vi "Main.vi"() -> ()   [LabVIEW 2014]
uses:
  TypeDefs/Errors.ctl
  <vilib>/Utility/file.llb/Read From Spreadsheet File (string).vi
  <vilib>/Waveform/DWDTOps.llb/DWDT Analog to Digital.vi
panel:
  out "Array":dbl[](array[numeric])
  out "Array 3":dbl[](array[numeric])
  out "Digital signals":cluster{dbl[], dbl[]}[](graph)
  out "digitsl signals":cluster{dbl[], dbl[]}(graph)
  in  "# of Files":i32=10
  out "# of rows":i32
  in  "File Locations":T1={"01 File Path"=path "C:/Users/502424328/Desktop/Ex Dish Inverter Board Data.csv", "02 File Path"=path "C:/Users/502424328/Desktop/Ex Dish Inverter Board Data.csv", "03 File Path"=path "C:/Users/502424328/Desktop/Ex Dish Inverter Board Data.csv", "04 File Path"=path "C:/Users/502424328/Desktop/Ex Dish Inverter Board Data.csv", "05 File Path"=path "C:/Users/502424328/Desktop/Ex Dish Inverter Board Data.csv", "06 File Path"=path "C:/Users/502424328/Desktop/Ex Dish Inverter Board Data.csv", "07 File Path"=path "C:/Users/502424328/Desktop/Ex Dish Inverter Board Data.csv", "08 File Path"=path "C:/Users/502424328/Desktop/Ex Dish Inverter Board Data.csv", "09 File Path"=path "C:/Users/502424328/Desktop/Ex Dish Inverter Board Data.csv", "10 File Path"=path "C:/Users/502424328/Desktop/Ex Dish Inverter Board Data.csv"}
  in  "Tab Control":T2(tab)
  out "Current (mA)":cluster{dbl[], dbl[]}(graph)
  out "Motor Type\n0 = MAIN\n1 = DRAIN":digitalwaveform(graph)
  out "XY Graph 10":cluster{dbl[], dbl[]}[](graph)
  out "Errors 1":T3
  out "XY Graph 9":cluster{dbl[], dbl[]}[](graph)
  out "Motor Type 2\n0 = MAIN\n1 = DRAIN 2":digitalwaveform(graph)
  out "Errors 2":T3
  out "Current 2 (mA)":cluster{dbl[], dbl[]}(graph)
  out "XY Graph 8":cluster{dbl[], dbl[]}[](graph)
  out "Motor Type 3\n0 = MAIN\n1 = DRAIN":digitalwaveform(graph)
  out "Errors 3":T3
  out "Current 3 (mA)":cluster{dbl[], dbl[]}(graph)
  out "XY Graph 7":cluster{dbl[], dbl[]}[](graph)
  out "Motor Type 4\n0 = MAIN\n1 = DRAIN":digitalwaveform(graph)
  out "Errors 4":T3
  out "Current 4 (mA)":cluster{dbl[], dbl[]}(graph)
  out "XY Graph 6":cluster{dbl[], dbl[]}[](graph)
  out "Motor Type 5\n0 = MAIN\n1 = DRAIN":digitalwaveform(graph)
  out "Errors 5":T3
  out "Current 5 (mA)":cluster{dbl[], dbl[]}(graph)
  out "Motor Type 6\n0 = MAIN\n1 = DRAIN":digitalwaveform(graph)
  out "Errors 6":T3
  out "Current 6 (mA)":cluster{dbl[], dbl[]}(graph)
  out "XY Graph 5":cluster{dbl[], dbl[]}[](graph)
  out "XY Graph 4":cluster{dbl[], dbl[]}[](graph)
  out "Motor Type 7\n0 = MAIN\n1 = DRAIN":digitalwaveform(graph)
  out "Errors 7":T3
  out "Current 7 (mA)":cluster{dbl[], dbl[]}(graph)
  out "XY Graph 3":cluster{dbl[], dbl[]}[](graph)
  out "Motor Type 8\n0 = MAIN\n1 = DRAIN":digitalwaveform(graph)
  out "Errors 8":T3
  out "Current 8 (mA)":cluster{dbl[], dbl[]}(graph)
  out "XY Graph 2":cluster{dbl[], dbl[]}[](graph)
  out "Motor Type 9\n0 = MAIN\n1 = DRAIN":digitalwaveform(graph)
  out "Errors 9":T3
  out "Current 9 (mA)":cluster{dbl[], dbl[]}(graph)
  out "XY Graph":cluster{dbl[], dbl[]}[](graph)
  out "Motor Type 10\n0 = MAIN\n1 = DRAIN":digitalwaveform(graph)
  out "Errors 10":T3
  out "Current 10 (mA)":cluster{dbl[], dbl[]}(graph)
  out "subarray":string[][](array[string])
  out "subarray 3":string[](array[string])
  in  "stop":bool
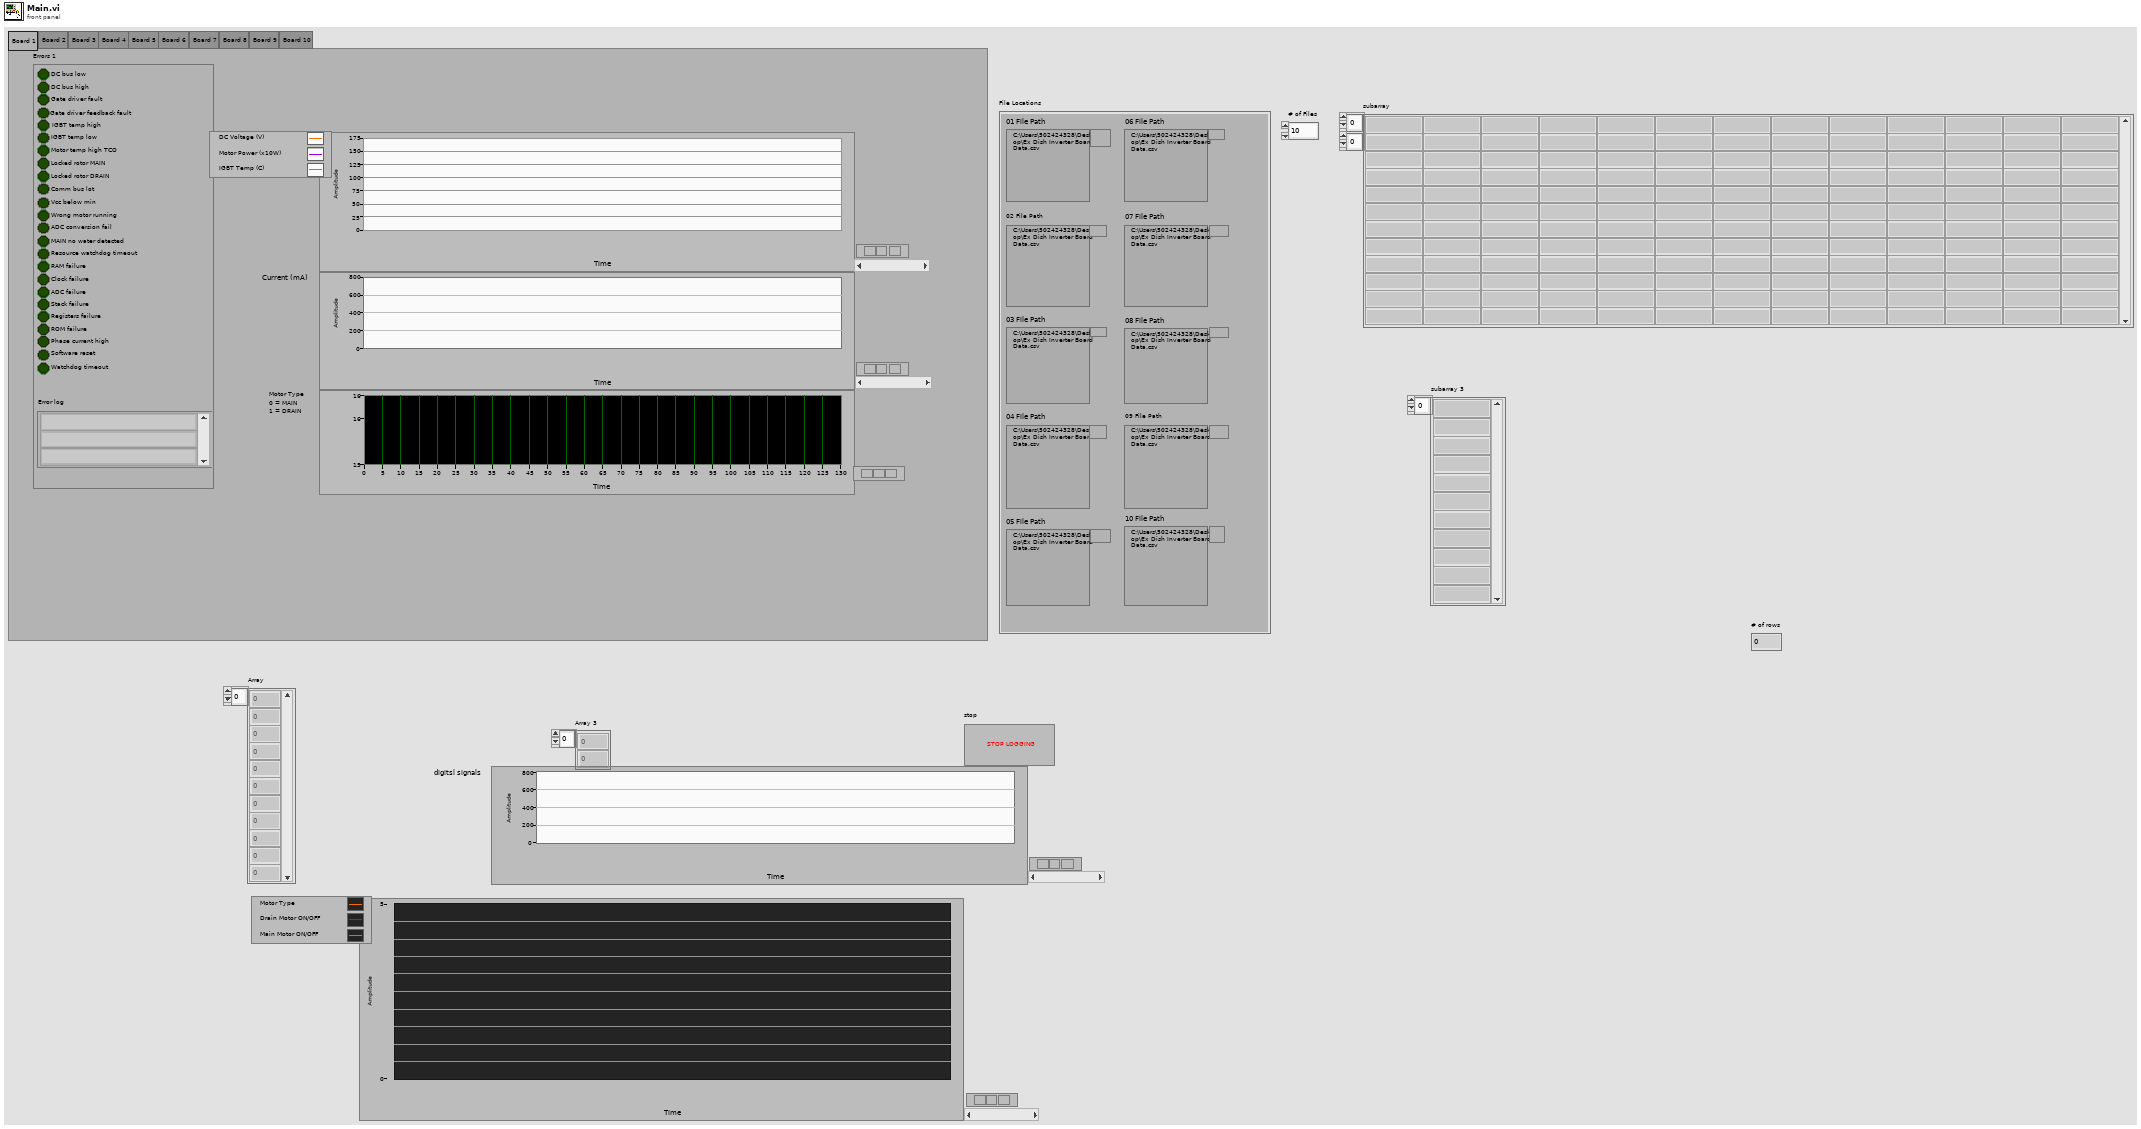
[diagram p1: front panel]
types:
  T1 = cluster{"01 File Path":path, "02 File Path":path, "03 File Path":path, "04 File Path":path, "05 File Path":path, "06 File Path":path, "07 File Path":path, "08 File Path":path, "09 File Path":path, "10 File Path":path}
  T2 = enum32{"Board 1", "Board 2", "Board 3", "Board 4", "Board 5", "Board 6", "Board 7", "Board 8", "Board 9", "Board 10"}
  T3 = typedef "Errors.ctl" = cluster{"DC bus low":bool, "DC bus high":bool, "Gate driver fault":bool, "Gate driver feedback fault":bool, "IGBT temp high":bool, "IGBT temp low":bool, "Motor temp high TCO":bool, "Locked rotor MAIN":bool, "Locked rotor DRAIN":bool, "Comm bus lot":bool, "Vcc below min":bool, "Wrong motor running":bool, "ADC conversion fail":bool, "MAIN no water detected":bool, "Resource watchdog timeout":bool, "RAM failure":bool, "Clock failure":bool, "ADC failure":bool, "Stack failure":bool, "Registers failure":bool, "ROM failure":bool, "Phase current high":bool, "Software reset":bool, "Watchdog timeout":bool, "Error log":string[]}
  T4 = cluster{"DC Bus Voltage":dbl, "Current RMS":dbl, "Motor Power":dbl, "IGBT Temp":u16, "Motor Type":u16, "Motor Power Sign":string, "Relay Position":u16, "ADC Count":dbl, "Recirculation Motor ON/OFF":u16, "Drain Motor ON/OFF":u16}
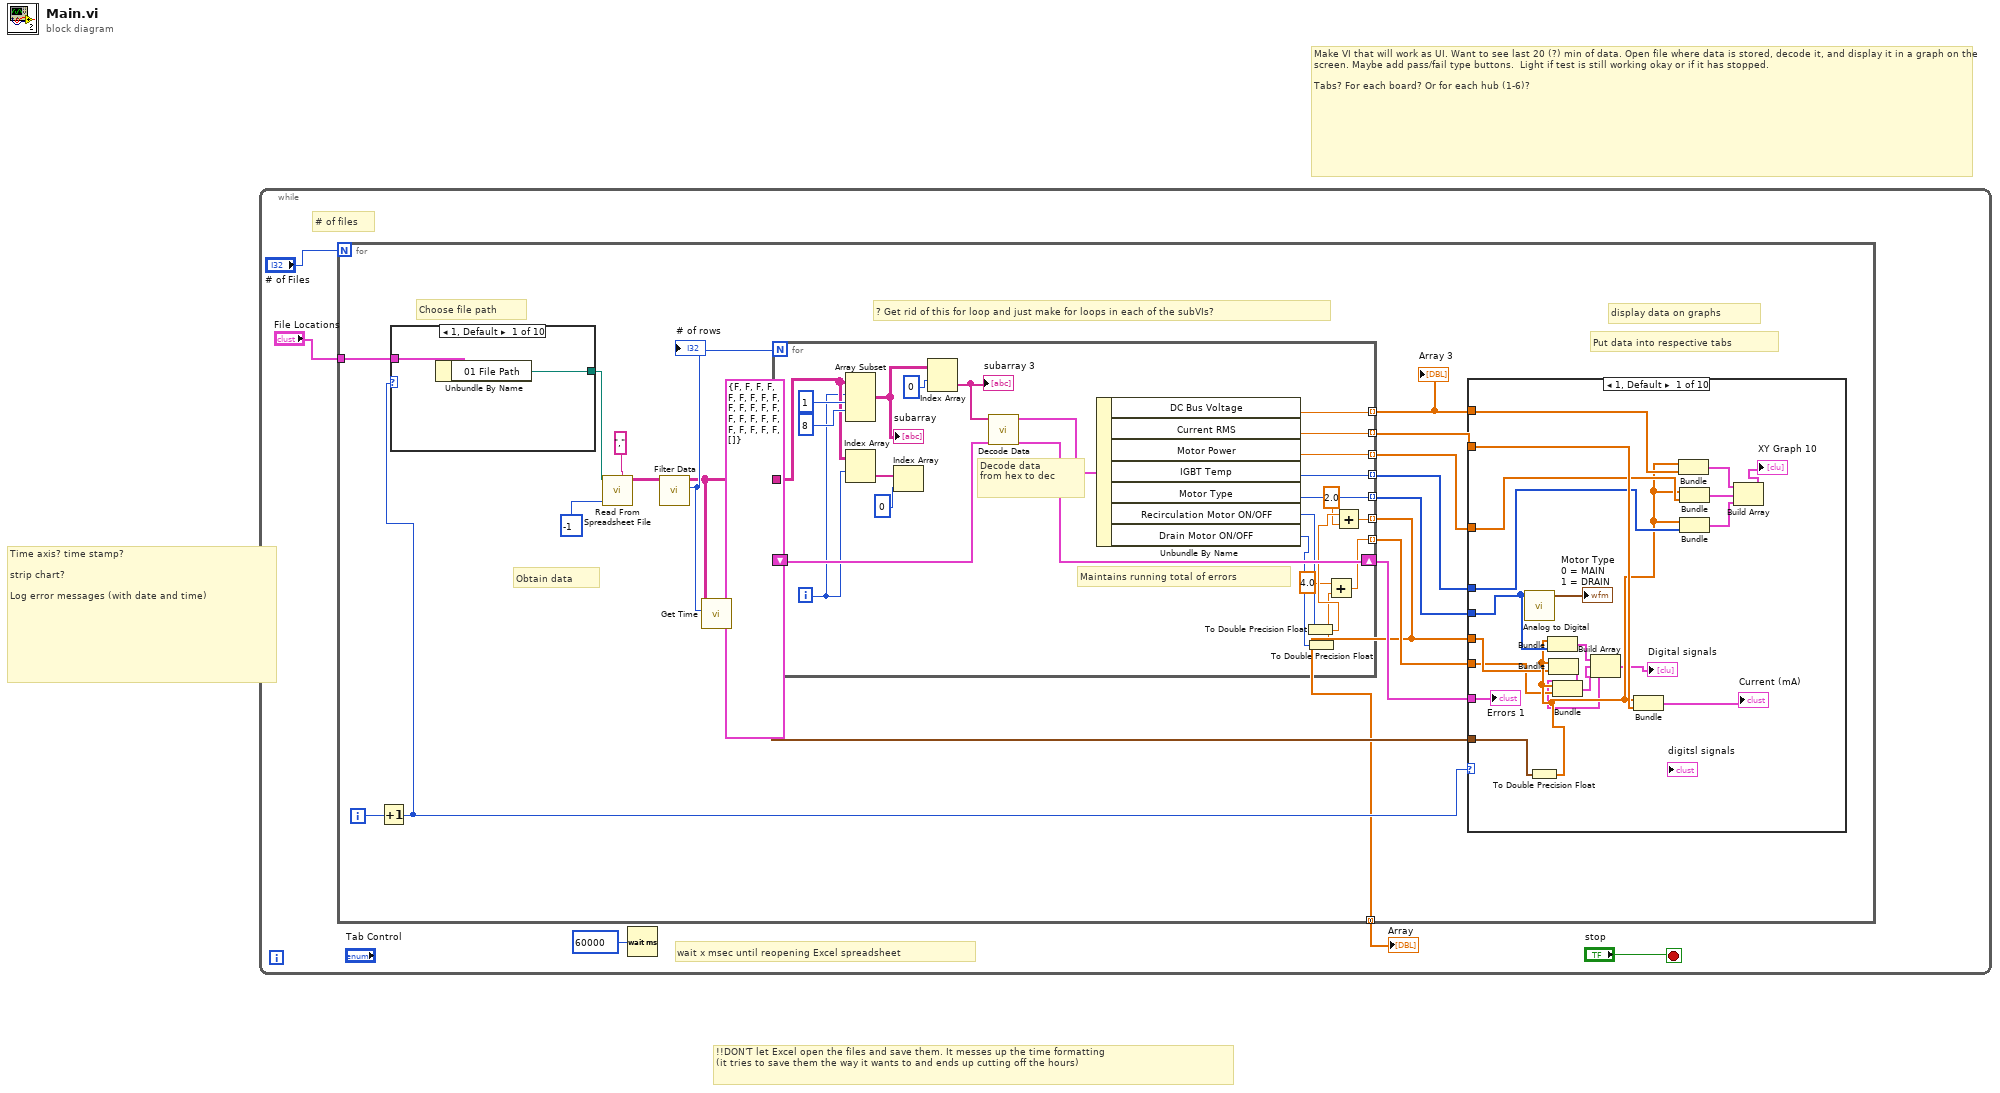
[diagram p0: block diagram]
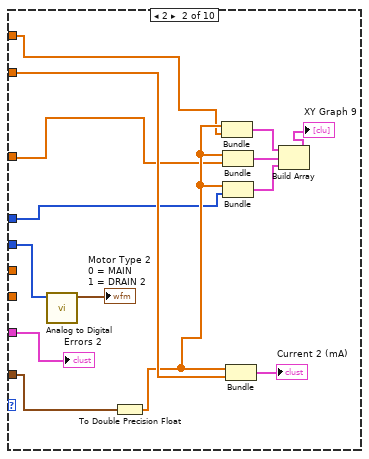
[diagram p2: hidden frame]
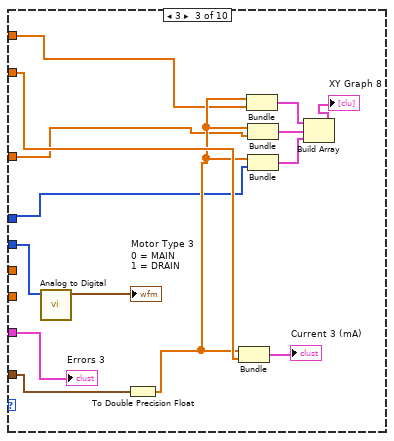
[diagram p3: hidden frame]
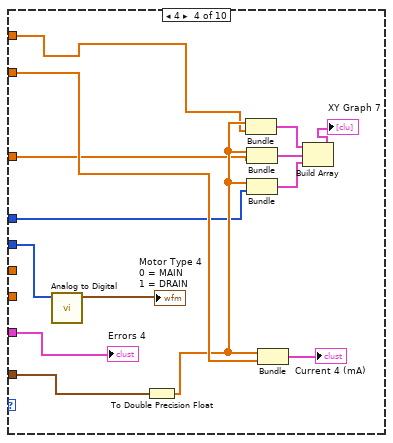
[diagram p4: hidden frame]
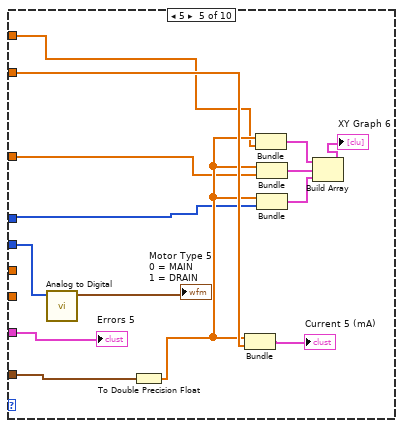
[diagram p5: hidden frame]
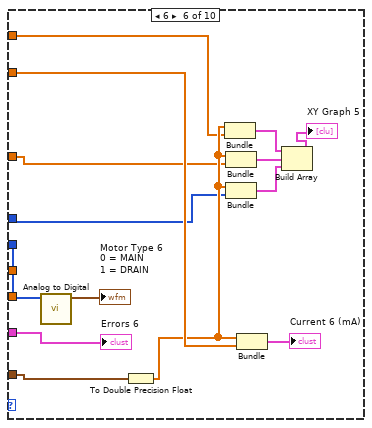
[diagram p6: hidden frame]
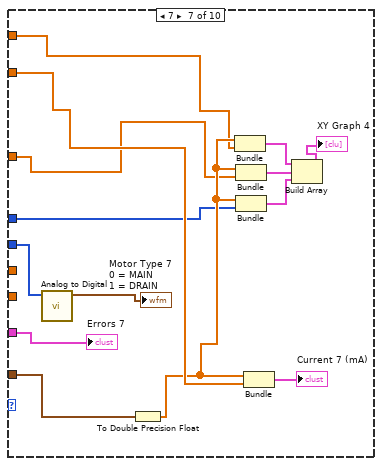
[diagram p7: hidden frame]
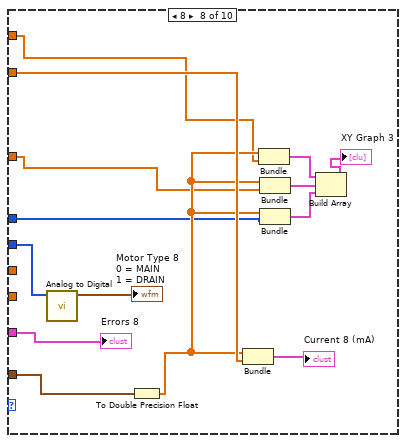
[diagram p8: hidden frame]
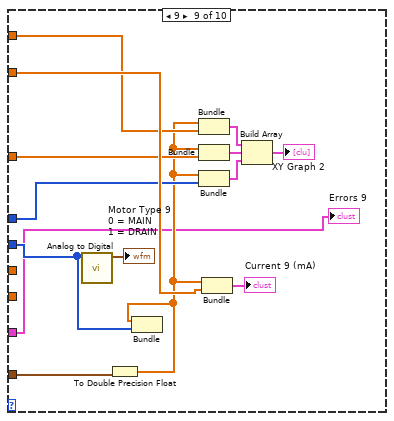
[diagram p9: hidden frame]
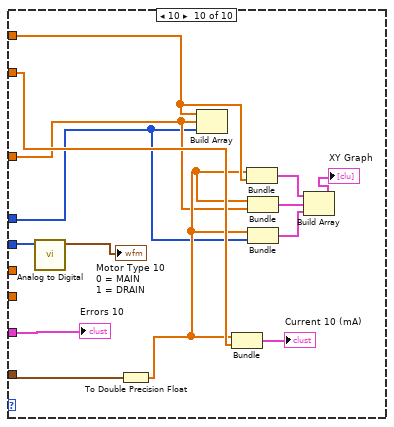
[diagram p10: hidden frame]
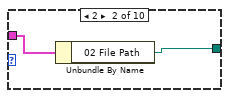
[diagram p11: hidden frame]
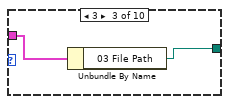
[diagram p12: hidden frame]
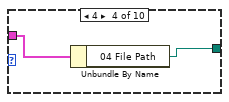
[diagram p13: hidden frame]
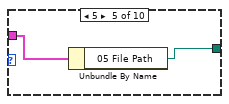
[diagram p14: hidden frame]
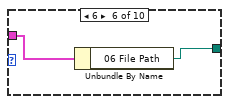
[diagram p15: hidden frame]
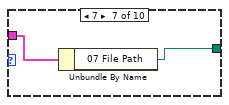
[diagram p16: hidden frame]
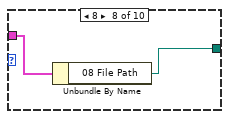
[diagram p17: hidden frame]
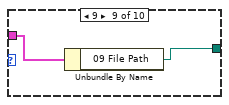
[diagram p18: hidden frame]
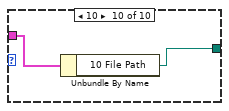
[diagram p19: hidden frame]
diagram:
  # "Time axis? time stamp?\n\nstrip chart?\n\nLog error messages (with date and time)"
  # "!!DON'T let Excel open the files and save them. It messes up the time formatting \n(it tries to save them the way it wants to and ends up cutting off the hours)"
  # "Make VI that will work as UI. Want to see last 20 (?) min of data. Open file where data is stored, decode it, and display it in a graph on the screen. Maybe add pass/fail type buttons.  Light if test is still working okay or if it has stopped. \n\nTabs? For each board? Or for each hub (1-6)?"
  n1 = while {
    stop <- "stop" stop-if-true
    # "# of files"
    # "wait x msec until reopening Excel spreadsheet"
    n2 = for {
      N: "# of Files" -> [_]
      tunnel: "File Locations" -> [w22]
      tunnel: [w6] -> w1 mode=concatenating
      i -> [w20]
      # "? Get rid of this for loop and just make for loops in each of the subVIs?"
      # "display data on graphs"
      # "Put data into respective tabs"
      # "Obtain data"
      # "Choose file path"
      n3 = Increment(x=w20) -> (x+1=w19:i32)
      n4 = case shown="1, Default" w19 {
        tunnel: w22 -> [w172 w174 w176 w178 w180 w182 w184 w186 w188 w190]
        tunnel: [w171 w173 w175 w177 w179 w181 w183 w185 w187 w189] -> w21
        frame 1, Default {
          n5 = Unbundle By Name(w172) -> ("01 File Path"=w171:path)
        }
        frame 2 {
          n6 = Unbundle By Name(w174) -> ("02 File Path"=w173:path)
        }
        frame 3 {
          n7 = Unbundle By Name(w176) -> ("03 File Path"=w175:path)
        }
        frame 4 {
          n8 = Unbundle By Name(w178) -> ("04 File Path"=w177:path)
        }
        frame 5 {
          n9 = Unbundle By Name(w180) -> ("05 File Path"=w179:path)
        }
        frame 6 {
          n10 = Unbundle By Name(w182) -> ("06 File Path"=w181:path)
        }
        frame 7 {
          n11 = Unbundle By Name(w184) -> ("07 File Path"=w183:path)
        }
        frame 8 {
          n12 = Unbundle By Name(w186) -> ("08 File Path"=w185:path)
        }
        frame 9 {
          n13 = Unbundle By Name(w188) -> ("09 File Path"=w187:path)
        }
        frame 10 {
          n14 = Unbundle By Name(w190) -> ("10 File Path"=w189:path)
        }
      }
      n15 = call-poly <vilib>:"Read From Spreadsheet File.vi"("delimiter (\\t)"="," ("delimiter (\\t)"), "number of rows (all:-1)"=-1, "file path (dialog if empty)"=w21) -> ("all rows"=w12:string[][])  [unwired: 4 in, 4 out]
      n16 = call "Filter Data.vi"("All Rows"=w12) -> ("element"=w11:i32, "new array"=w10:string[][])  [unwired: 9 in]
      "# of rows" <- w11
      n17 = call "Get Time.vi"("# of rows"=w11, "Data row"=w10) -> ("Time array"=w9:timestamp[])  [unwired: 9 in]
      n18 = for {
        N: w11 -> [_]
        tunnel: [w211] -> w16 mode=indexing
        tunnel: [w210] -> w18 mode=indexing
        tunnel: [w209] -> w17 mode=indexing
        tunnel: [w208] -> w15 mode=indexing
        tunnel: [w207] -> w14 mode=indexing
        shift-right: [w206] -> w13
        shift-left: T3 {"DC bus low"=FALSE, "DC bus high"=FALSE, "Gate driver fault"=FALSE, "Gate driver feedback fault"=FALSE, "IGBT temp high"=FALSE, "IGBT temp low"=FALSE, "Motor temp high TCO"=FALSE, "Locked rotor MAIN"=FALSE, "Locked rotor DRAIN"=FALSE, "Comm bus lot"=FALSE, "Vcc below min"=FALSE, "Wrong motor running"=FALSE, "ADC conversion fail"=FALSE, "MAIN no water detected"=FALSE, "Resource watchdog timeout"=FALSE, "RAM failure"=FALSE, "Clock failure"=FALSE, "ADC failure"=FALSE, "Stack failure"=FALSE, "Registers failure"=FALSE, "ROM failure"=FALSE, "Phase current high"=FALSE, "Software reset"=FALSE, "Watchdog timeout"=FALSE, "Error log"=[]} ("Errors Out") -> [w205]
        tunnel: w10 -> [w202]
        tunnel: [w198] -> w6 mode=indexing
        tunnel: [w197] -> w7 mode=indexing
        i -> [w199]
        # "Maintains running total of errors"
        # "Decode data\nfrom hex to dec"
        n19 = Array Subset(array=w202, index (row)=w199, length (row)=1 ("length"), index (col)=8 ("index")) -> (w213:string[][])  [unwired: 1 in]
        "subarray" <- w213
        n20 = Index Array(array=w202, index (row)=w199) -> (element=w201:string[])  [unwired: 1 in]
        n21 = Index Array(array=w201, index=0) -> ()  [unwired: 1 out]
        n22 = Index Array(array=w213, index (row)=0 ("disabled index (col)")) -> (element=w203:string[])  [unwired: 1 in]
        "subarray 3" <- w203
        n23 = call "Decode Data.vi"("Errors In"=w205, "Data Array"=w203) -> ("Errors Out"=w206:T3, "logData Out"=w204:T4)  [unwired: 8 in]
        n24 = Unbundle By Name(w204) -> ("DC Bus Voltage"=w211:dbl, "Current RMS"=w210:dbl, "Motor Power"=w209:dbl, "IGBT Temp"=w208:u16, "Motor Type"=w207:u16, "Recirculation Motor ON/OFF"=w196:u16, "Drain Motor ON/OFF"=w193:u16)
        n25 = To Double Precision Float(number=w196) -> (double precision float=w195:dbl)
        n26 = To Double Precision Float(number=w193) -> (double precision float=w192:dbl)
        n27 = Add(x=4.0, y=w192) -> (x+y=w197:dbl)
        n28 = Add(x=w195, y=2.0) -> (x+y=w198:dbl)
      }
      "Array 3" <- w16
      n29 = case shown="1, Default" w19 {
        tunnel: w18 -> [w42 w54 w68 w82 w96 w110 w124 w138 w155 w166]
        tunnel: w17 -> [w34 w46 w60 w73 w88 w102 w116 w130 w150 w162]
        tunnel: w16 -> [w35 w47 w61 w75 w89 w103 w117 w131 w151 w164]
        tunnel: w15 -> [w33 w45 w59 w74 w87 w101 w115 w129 w149 w161]
        tunnel: w14 -> [w32 w58 w72 w86 w100 w114 w128 w142 w146 w170]
        tunnel: w13 -> [w43 w56 w70 w84 w98 w112 w126 w140 w145 w168]
        tunnel: w9 -> [w41 w55 w69 w83 w97 w111 w125 w139 w156 w167]
        tunnel: w6 -> [w30 _ _ _ _ _ _ _ _ _]
        tunnel: w7 -> [w29 _ _ _ _ _ _ _ _ _]
        frame 1, Default {
          n30 = call-poly <vilib>:"Analog to Digital.vi"("analog waveform"=w32) -> ("digital waveform"=→"Motor Type\n0 = MAIN\n1 = DRAIN":digitalwaveform)  [unwired: 7 in, 3 out]
          n31 = To Double Precision Float(number=w41) -> (double precision float=w31:dbl[])
          n32 = Bundle(w31, w32) -> (w28:cluster{dbl[], u16[]})  [unwired: 1 in]
          n33 = Bundle(w31, w30) -> (w25:cluster{dbl[], dbl[]})  [unwired: 1 in]
          n34 = Bundle(w31, w29) -> (w26:cluster{dbl[], dbl[]})  [unwired: 1 in]
          n35 = Build Array(w28, w26, w25) -> (→"Digital signals":cluster{dbl[], dbl[]}[])
          n36 = Bundle(w31, w42) -> (→"Current (mA)":cluster{dbl[], dbl[]})  [unwired: 1 in]
          n37 = Bundle(w31, w35) -> (w39:cluster{dbl[], dbl[]})  [unwired: 1 in]
          n38 = Bundle(w31, w34) -> (w38:cluster{dbl[], dbl[]})  [unwired: 1 in]
          n39 = Bundle(w31, w33) -> (w37:cluster{dbl[], u16[]})  [unwired: 1 in]
          n40 = Build Array(w39, w38, w37) -> (→"XY Graph 10":cluster{dbl[], dbl[]}[])
          "Errors 1" <- w43
        }
        frame 2 {
          n41 = call-poly <vilib>:"Analog to Digital.vi"("analog waveform"=w58) -> ("digital waveform"=→"Motor Type 2\n0 = MAIN\n1 = DRAIN 2":digitalwaveform)  [unwired: 7 in, 3 out]
          n42 = To Double Precision Float(number=w55) -> (double precision float=w48:dbl[])
          n43 = Bundle(w48, w47) -> (w52:cluster{dbl[], dbl[]})  [unwired: 1 in]
          n44 = Bundle(w48, w46) -> (w51:cluster{dbl[], dbl[]})  [unwired: 1 in]
          n45 = Bundle(w48, w45) -> (w50:cluster{dbl[], u16[]})  [unwired: 1 in]
          n46 = Bundle(w48, w54) -> (→"Current 2 (mA)":cluster{dbl[], dbl[]})  [unwired: 1 in]
          n47 = Build Array(w52, w51, w50) -> (→"XY Graph 9":cluster{dbl[], dbl[]}[])
          "Errors 2" <- w56
        }
        frame 3 {
          n48 = call-poly <vilib>:"Analog to Digital.vi"("analog waveform"=w72) -> ("digital waveform"=→"Motor Type 3\n0 = MAIN\n1 = DRAIN":digitalwaveform)  [unwired: 7 in, 3 out]
          n49 = To Double Precision Float(number=w69) -> (double precision float=w62:dbl[])
          n50 = Bundle(w62, w68) -> (→"Current 3 (mA)":cluster{dbl[], dbl[]})  [unwired: 1 in]
          n51 = Bundle(w62, w61) -> (w66:cluster{dbl[], dbl[]})  [unwired: 1 in]
          n52 = Bundle(w62, w60) -> (w65:cluster{dbl[], dbl[]})  [unwired: 1 in]
          n53 = Bundle(w62, w59) -> (w64:cluster{dbl[], u16[]})  [unwired: 1 in]
          n54 = Build Array(w66, w65, w64) -> (→"XY Graph 8":cluster{dbl[], dbl[]}[])
          "Errors 3" <- w70
        }
        frame 4 {
          n55 = call-poly <vilib>:"Analog to Digital.vi"("analog waveform"=w86) -> ("digital waveform"=→"Motor Type 4\n0 = MAIN\n1 = DRAIN":digitalwaveform)  [unwired: 7 in, 3 out]
          n56 = To Double Precision Float(number=w83) -> (double precision float=w76:dbl[])
          n57 = Bundle(w76, w75) -> (w80:cluster{dbl[], dbl[]})  [unwired: 1 in]
          n58 = Bundle(w76, w73) -> (w79:cluster{dbl[], dbl[]})  [unwired: 1 in]
          n59 = Bundle(w76, w74) -> (w78:cluster{dbl[], u16[]})  [unwired: 1 in]
          n60 = Bundle(w76, w82) -> (→"Current 4 (mA)":cluster{dbl[], dbl[]})  [unwired: 1 in]
          n61 = Build Array(w80, w79, w78) -> (→"XY Graph 7":cluster{dbl[], dbl[]}[])
          "Errors 4" <- w84
        }
        frame 5 {
          n62 = call-poly <vilib>:"Analog to Digital.vi"("analog waveform"=w100) -> ("digital waveform"=→"Motor Type 5\n0 = MAIN\n1 = DRAIN":digitalwaveform)  [unwired: 7 in, 3 out]
          n63 = To Double Precision Float(number=w97) -> (double precision float=w90:dbl[])
          n64 = Bundle(w90, w96) -> (→"Current 5 (mA)":cluster{dbl[], dbl[]})  [unwired: 1 in]
          n65 = Bundle(w90, w89) -> (w94:cluster{dbl[], dbl[]})  [unwired: 1 in]
          n66 = Bundle(w90, w88) -> (w93:cluster{dbl[], dbl[]})  [unwired: 1 in]
          n67 = Bundle(w90, w87) -> (w92:cluster{dbl[], u16[]})  [unwired: 1 in]
          n68 = Build Array(w94, w93, w92) -> (→"XY Graph 6":cluster{dbl[], dbl[]}[])
          "Errors 5" <- w98
        }
        frame 6 {
          n69 = call-poly <vilib>:"Analog to Digital.vi"("analog waveform"=w114) -> ("digital waveform"=→"Motor Type 6\n0 = MAIN\n1 = DRAIN":digitalwaveform)  [unwired: 7 in, 3 out]
          n70 = To Double Precision Float(number=w111) -> (double precision float=w104:dbl[])
          n71 = Bundle(w104, w103) -> (w108:cluster{dbl[], dbl[]})  [unwired: 1 in]
          n72 = Bundle(w104, w102) -> (w107:cluster{dbl[], dbl[]})  [unwired: 1 in]
          n73 = Bundle(w104, w101) -> (w106:cluster{dbl[], u16[]})  [unwired: 1 in]
          n74 = Bundle(w104, w110) -> (→"Current 6 (mA)":cluster{dbl[], dbl[]})  [unwired: 1 in]
          n75 = Build Array(w108, w107, w106) -> (→"XY Graph 5":cluster{dbl[], dbl[]}[])
          "Errors 6" <- w112
        }
        frame 7 {
          n76 = call-poly <vilib>:"Analog to Digital.vi"("analog waveform"=w128) -> ("digital waveform"=→"Motor Type 7\n0 = MAIN\n1 = DRAIN":digitalwaveform)  [unwired: 7 in, 3 out]
          n77 = To Double Precision Float(number=w125) -> (double precision float=w118:dbl[])
          n78 = Bundle(w118, w117) -> (w122:cluster{dbl[], dbl[]})  [unwired: 1 in]
          n79 = Bundle(w118, w116) -> (w121:cluster{dbl[], dbl[]})  [unwired: 1 in]
          n80 = Bundle(w118, w115) -> (w120:cluster{dbl[], u16[]})  [unwired: 1 in]
          n81 = Bundle(w118, w124) -> (→"Current 7 (mA)":cluster{dbl[], dbl[]})  [unwired: 1 in]
          n82 = Build Array(w122, w121, w120) -> (→"XY Graph 4":cluster{dbl[], dbl[]}[])
          "Errors 7" <- w126
        }
        frame 8 {
          n83 = call-poly <vilib>:"Analog to Digital.vi"("analog waveform"=w142) -> ("digital waveform"=→"Motor Type 8\n0 = MAIN\n1 = DRAIN":digitalwaveform)  [unwired: 7 in, 3 out]
          n84 = To Double Precision Float(number=w139) -> (double precision float=w132:dbl[])
          n85 = Bundle(w132, w138) -> (→"Current 8 (mA)":cluster{dbl[], dbl[]})  [unwired: 1 in]
          n86 = Bundle(w132, w131) -> (w136:cluster{dbl[], dbl[]})  [unwired: 1 in]
          n87 = Bundle(w132, w130) -> (w135:cluster{dbl[], dbl[]})  [unwired: 1 in]
          n88 = Bundle(w132, w129) -> (w134:cluster{dbl[], u16[]})  [unwired: 1 in]
          n89 = Build Array(w136, w135, w134) -> (→"XY Graph 3":cluster{dbl[], dbl[]}[])
          "Errors 8" <- w140
        }
        frame 9 {
          n90 = call-poly <vilib>:"Analog to Digital.vi"("analog waveform"=w146) -> ("digital waveform"=→"Motor Type 9\n0 = MAIN\n1 = DRAIN":digitalwaveform)  [unwired: 7 in, 3 out]
          n91 = To Double Precision Float(number=w156) -> (double precision float=w147:dbl[])
          n92 = Bundle(w147, w146) -> ()  [unwired: 1 in, 1 out]
          n93 = Bundle(w147, w151) -> (w153:cluster{dbl[], dbl[]})  [unwired: 1 in]
          n94 = Bundle(w147, w150) -> (w152:cluster{dbl[], dbl[]})  [unwired: 1 in]
          n95 = Bundle(w147, w149) -> (w144:cluster{dbl[], u16[]})  [unwired: 1 in]
          n96 = Bundle(w147, w155) -> (→"Current 9 (mA)":cluster{dbl[], dbl[]})  [unwired: 1 in]
          n97 = Build Array(w153, w152, w144) -> (→"XY Graph 2":cluster{dbl[], dbl[]}[])
          "Errors 9" <- w145
        }
        frame 10 {
          n98 = call-poly <vilib>:"Analog to Digital.vi"("analog waveform"=w170) -> ("digital waveform"=→"Motor Type 10\n0 = MAIN\n1 = DRAIN":digitalwaveform)  [unwired: 7 in, 3 out]
          n99 = To Double Precision Float(number=w167) -> (double precision float=w163:dbl[])
          n100 = Build Array(w164, w162, w161) -> ()  [unwired: 1 out]
          n101 = Bundle(w163, w166) -> (→"Current 10 (mA)":cluster{dbl[], dbl[]})  [unwired: 1 in]
          n102 = Bundle(w163, w164) -> (w160:cluster{dbl[], dbl[]})  [unwired: 1 in]
          n103 = Bundle(w163, w162) -> (w159:cluster{dbl[], dbl[]})  [unwired: 1 in]
          n104 = Bundle(w163, w161) -> (w158:cluster{dbl[], u16[]})  [unwired: 1 in]
          n105 = Build Array(w160, w159, w158) -> (→"XY Graph":cluster{dbl[], dbl[]}[])
          "Errors 10" <- w168
        }
      }
    }
    "Array" <- w1
    n106 = Wait (ms)(milliseconds to wait=u32 60000) -> ()  [unwired: 1 out]
  }
